vi "PIXMAP.vi"(7 "IV Folder Path":path, 8 "error in (no error)":errorcluster, 9 "Height":i16, 10 "Width":i16, 11 "2D Pixmap":u32[][](array[numeric])) -> (0 "error out":errorcluster)   [LabVIEW 2023]
panel:
  out "Pixmap.bin":u32[](array[numeric])
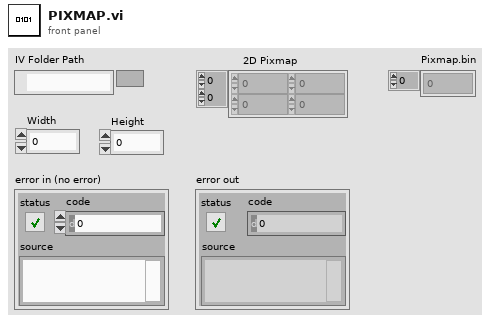
[diagram p1: front panel]
types:
  T1 = enum16{"big-endian, network order", "native, host order", "little-endian"}
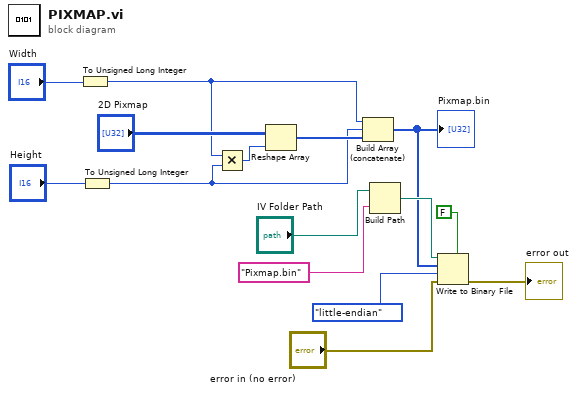
[diagram p0: block diagram]
diagram:
  n1 = To Unsigned Long Integer(number="Width") -> (unsigned 32bit integer=w10:u32)
  n2 = To Unsigned Long Integer(number="Height") -> (unsigned 32bit integer=w9:u32)
  n3 = Multiply(x=w10, y=w9) -> (x*y=w11:u32)
  n4 = Reshape Array("2D Pixmap", w11) -> (w12:u32[])
  n5 = Build Array (concatenate)(w10, w9, w12) -> (w3:u32[])
  "Pixmap.bin" <- w3
  n6 = Build Path(base path="IV Folder Path", name or relative path="Pixmap.bin") -> (appended path=w6:path)
  n7 = Write to Binary File(file (use dialog)=w6, data=w3, error in="error in (no error)", 5:FALSE, 9:T1."little-endian" ("byte order (0:big-endian, network order)")) -> (error out=→"error out":errorcluster)  [unwired: 1 in, 2 out]
